vi "F510-X.vi"(8 "error in (no error)":errorcluster, 10 "Deadzone Scale Cluster":cluster{"Scale":dbl, "Deadzone":dbl}={"Scale"=1.0, "Deadzone"=0.1}, 11 "refnum name":string) -> (0 "error out":errorcluster, 1 "Right Stick":cluster{"X":dbl, "Y":dbl}, 2 "Left Stick":cluster{"X":dbl, "Y":dbl}, 3 "JoystickDevRef":T2, 4 "Buttons":T1, 5 "Triggers":cluster{"Left":dbl, "Right":dbl}, 6 "D-Pad Buttons":T4)   [LabVIEW 2015]
uses:
  <vilib>/Rock Robotics/WPI/Joystick/WPI_JoystickDevRef.ctl
  <vilib>/Rock Robotics/WPI/Joystick/WPI_JoystickDeviceEnum.ctl
  <vilib>/Rock Robotics/WPI/Utilities/WPI_GetSetVariantRefNum.vi
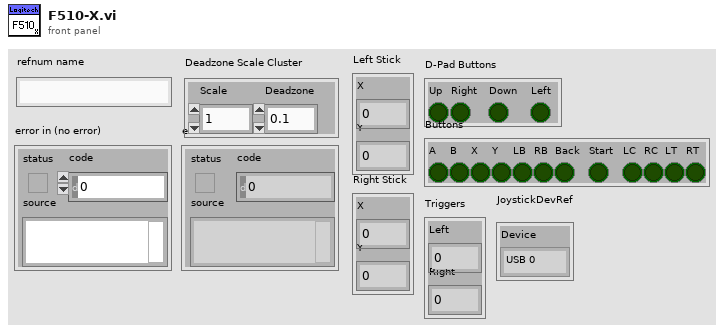
[diagram p1: front panel]
types:
  T1 = cluster{"A":bool, "B":bool, "X":bool, "Y":bool, "LB":bool, "RB":bool, "Back":bool, "Start":bool, "LC":bool, "RC":bool, "LT":bool, "RT":bool}
  T2 = typedef "WPI_JoystickDevRef.ctl" = cluster{"Device":T3}
  T3 = typedef "WPI_JoystickDeviceEnum.ctl" = enum16{"USB 0", "USB 1", "USB 2", "USB 3", "USB 4", "USB 5"}
  T4 = cluster{"Up":bool, "Right":bool, "Down":bool, "Left":bool}
  T5 = cluster{"[0]":dbl, "[1]":dbl, "[2]":dbl, "[3]":dbl, "[4]":dbl, "[5]":dbl}
  T6 = cluster{"Buttons[0]":bool, "Buttons[1]":bool, "Buttons[2]":bool, "Buttons[3]":bool, "Buttons[4]":bool, "Buttons[5]":bool, "Buttons[6]":bool, "Buttons[7]":bool, "Buttons[8]":bool, "Buttons[9]":bool}
  T7 = cluster{"Up":bool, "Down":bool, "Left":bool, "Right":bool}[]
  T8 = cluster{"Up":bool, "Down":bool, "Left":bool, "Right":bool}
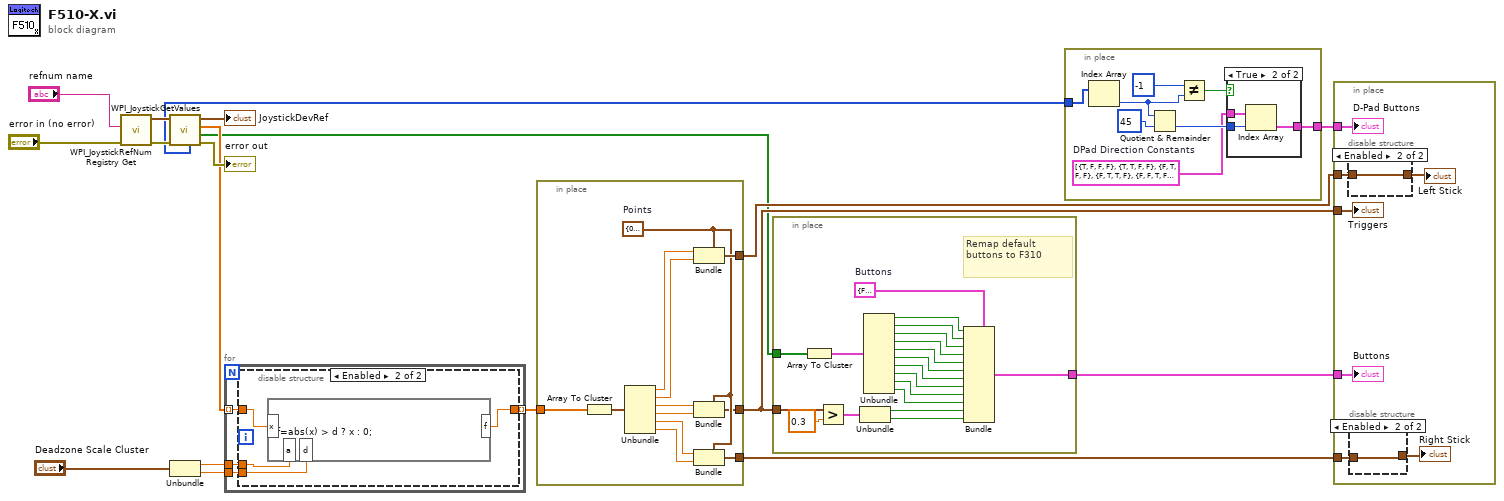
[diagram p0: block diagram]
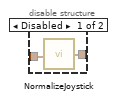
[diagram p2: hidden frame]
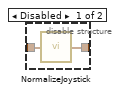
[diagram p3: hidden frame]
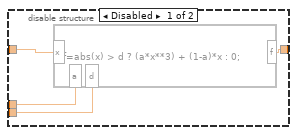
[diagram p5: hidden frame]
diagram:
  n1 = call <vilib>:"WPI_JoystickRefNum Registry Get.vi"("error in (no error)"="error in (no error)", "refnum name"="refnum name") -> ("error out"=w15:errorcluster, "JoystickDevRef"=w16:T2)  [unwired: 8 in]
  n2 = call <vilib>:"WPI_JoystickGetValues.vi"("error in (no error)"=w15, "JoystickDevRef"=w16) -> ("error out"=→"error out":errorcluster, "Buttons"=w2:bool[], "Axes"=w13:dbl[], "JoystickDevRef"=→"JoystickDevRef":T2, "POVs"=w6:i16[])  [unwired: 5 in]
  n3 = Unbundle("Deadzone Scale Cluster") -> ("Scale"=w11:dbl, "Deadzone"=w10:dbl)
  n4 = for {
    tunnel: w13 -> [w22] mode=indexing
    tunnel: w11 -> [w21]
    tunnel: w10 -> [w20]
    tunnel: [w19] -> w9 mode=indexing
    n5 = disable-structure shown="Enabled" {
      disable-tunnel: w22 -> [w26 w28]
      disable-tunnel: w21 -> [w25 w30]
      disable-tunnel: w20 -> [w24 w29]
      disable-tunnel: [w23 w27] -> w19
      frame Disabled {
        n6 = formula code="f=abs(x) > d ? (a*x**3) + (1-a)*x : 0;"("x"=w26, "d"=w24, "a"=w25) -> ("f"=w23:dbl)
      }
      frame Enabled {
        n7 = formula code="f=abs(x) > d ? x : 0;"("x"=w28, "d"=w29, "a"=w30) -> ("f"=w27:dbl)
      }
    }
  }
  n8 = in-place {
    in-place-border: w9 -> [w39]
    in-place-border: [w35] -> w7
    in-place-border: [w38] -> w8
    in-place-border: [w33] -> w5
    w34 = cluster{"X":dbl, "Y":dbl} {"X"=0.0, "Y"=0.0}  # Points
    n9 = Array To Cluster(array=w39) -> (cluster=w42:T5)
    n10 = Unbundle(w42) -> ("[0]"=w40:dbl, "[1]"=w41:dbl, "[2]"=w32:dbl, "[3]"=w31:dbl, "[4]"=w37:dbl, "[5]"=w36:dbl)
    n11 = Bundle(cluster=w34, "X"=w40, "Y"=w41) -> (w38:cluster{"X":dbl, "Y":dbl})
    n12 = Bundle(cluster=w34, "X"=w32, "Y"=w31) -> (w33:cluster{"X":dbl, "Y":dbl})
    n13 = Bundle(cluster=w34, "X"=w37, "Y"=w36) -> (w35:cluster{"X":dbl, "Y":dbl})
  }
  n14 = in-place {
    in-place-border: w2 -> [w52]
    in-place-border: [w54] -> w1
    in-place-border: w5 -> [w47]
    w61 = T1 {"A"=FALSE, "B"=FALSE, "X"=FALSE, "Y"=FALSE, "LB"=FALSE, "RB"=FALSE, "Back"=FALSE, "Start"=FALSE, "LC"=FALSE, "RC"=FALSE, "LT"=FALSE, "RT"=FALSE}  # Buttons
    # "Remap default\nbuttons to F310"
    n15 = Array To Cluster(array=w52) -> (cluster=w53:T6)
    n16 = Greater?(x=w47, y=0.3) -> (0:w45:cluster{"X":bool, "Y":bool})
    n17 = Unbundle(w45) -> ("X"=w44:bool, "Y"=w43:bool)
    n18 = Unbundle(w53) -> ("Buttons[0]"=w60:bool, "Buttons[1]"=w59:bool, "Buttons[2]"=w58:bool, "Buttons[3]"=w57:bool, "Buttons[4]"=w56:bool, "Buttons[5]"=w55:bool, "Buttons[6]"=w51:bool, "Buttons[7]"=w50:bool, "Buttons[8]"=w49:bool, "Buttons[9]"=w48:bool)
    n19 = Bundle(cluster=w61, "A"=w60, "B"=w59, "X"=w58, "Y"=w57, "LB"=w56, "RB"=w55, "Back"=w51, "Start"=w50, "LC"=w49, "RC"=w48, "LT"=w44, "RT"=w43) -> (w54:T1)
  }
  n20 = in-place {
    in-place-border: w6 -> [w69]
    in-place-border: [w64] -> w4
    w65 = T7 [{"Up"=TRUE, "Down"=FALSE, "Left"=FALSE, "Right"=FALSE}, {"Up"=TRUE, "Down"=TRUE, "Left"=FALSE, "Right"=FALSE}, {"Up"=FALSE, "Down"=TRUE, "Left"=FALSE, "Right"=FALSE}, {"Up"=FALSE, "Down"=TRUE, "Left"=TRUE, "Right"=FALSE}, {"Up"=FALSE, "Down"=FALSE, "Left"=TRUE, "Right"=FALSE}, {"Up"=FALSE, "Down"=FALSE, "Left"=TRUE, "Right"=TRUE}, {"Up"=FALSE, "Down"=FALSE, "Left"=FALSE, "Right"=TRUE}, {"Up"=TRUE, "Down"=FALSE, "Left"=FALSE, "Right"=TRUE}]  # DPad Direction Constants
    n21 = Index Array(array=w69) -> (element=w63:i16)  [unwired: 1 in]
    n22 = Quotient & Remainder(x=w63, y=u16 45) -> (floor(x/y)=w67:u16)  [unwired: 1 out]
    n23 = Not Equal?(x=i16 -1, y=w63) -> (x != y?=w66:bool)
    n24 = case shown="True" w66 {
      tunnel: w67 -> [_ w72]
      tunnel: w65 -> [_ w71]
      tunnel: [_ w70] -> w64
      frame False {
      }
      frame True {
        n25 = Index Array(array=w71, index=w72) -> (element=w70:T8)
      }
    }
  }
  n26 = in-place {
    in-place-border: w8 -> [w76]
    in-place-border: w7 -> [w74]
    in-place-border: w5 -> [w79]
    in-place-border: w4 -> [w78]
    in-place-border: w1 -> [w77]
    n27 = disable-structure shown="Enabled" {
      disable-tunnel: w76 -> [w84 w85]
      disable-tunnel: [w83 w85] -> w75
      frame Disabled {
        n28 = call "NormalizeJoystick.vi"("joystick"=w84) -> ("normalized joystick"=w83:cluster{"x":dbl, "y":dbl})
      }
      frame Enabled {
      }
    }
    "Left Stick" <- w75
    n29 = disable-structure shown="Enabled" {
      disable-tunnel: w74 -> [w81 w82]
      disable-tunnel: [w80 w82] -> w73
      frame Disabled {
        n30 = call "NormalizeJoystick.vi"("joystick"=w81) -> ("normalized joystick"=w80:cluster{"x":dbl, "y":dbl})
      }
      frame Enabled {
      }
    }
    "Right Stick" <- w73
    "Triggers" <- w79
    "D-Pad Buttons" <- w78
    "Buttons" <- w77
  }
